vi "pid.vi"(0 "目标":dbl, 1 "当前":dbl, 2 "kp":dbl, 3 "ki":dbl, 4 "kd":dbl, 6 "重置积分":bool) -> (5 "out":dbl)   [LabVIEW 2022 SP3]
panel:
  out "pid微分":dbl
  out "pid积分":dbl
  out "d":dbl
  out "p":dbl
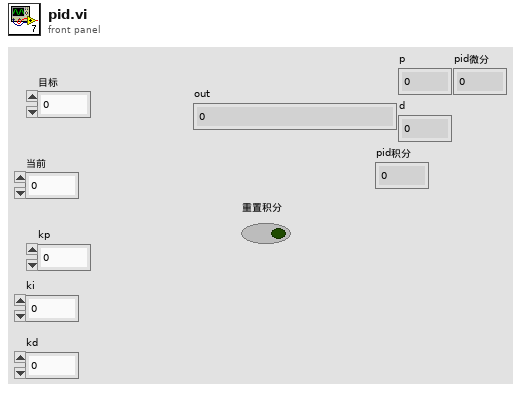
[diagram p1: front panel]
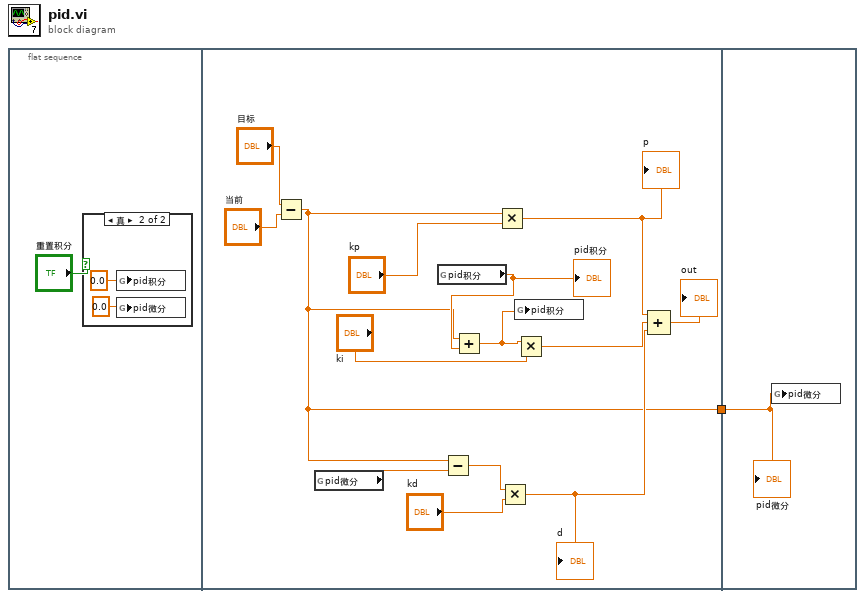
[diagram p0: block diagram]
diagram:
  n1 = flat-sequence {
    tunnel: [w5] -> w1
    tunnel: w1 -> [w19]
    frame #0 {
      n2 = case shown="真" "重置积分" {
        frame False {
        }
        frame True {
          n3 = global write "全局 1.vi" "pid积分"(0.0 ("pid积分")) -> ()
          n4 = global write "全局 1.vi" "pid微分"(0.0 ("pid积分")) -> ()
        }
      }
    }
    frame #1 {
      n5 = Subtract(x="目标", y="当前") -> (x-y=w5:dbl)
      n6 = global read "全局 1.vi" "pid微分"() -> (w6:dbl)
      n7 = global read "全局 1.vi" "pid积分"() -> (w18:dbl)
      "pid积分" <- w18
      n8 = Subtract(x=w5, y=w6) -> (x-y=w11:dbl)
      n9 = Add(x=w5, y=w18) -> (x+y=w17:dbl)
      n10 = Multiply(x=w5, y="kp") -> (x*y=w13:dbl)
      "p" <- w13
      n11 = Multiply(x=w11, y="kd") -> (x*y=w15:dbl)
      "d" <- w15
      n12 = global write "全局 1.vi" "pid积分"(w17) -> ()
      n13 = Multiply(x=w17, y="ki") -> (x*y=w14:dbl)
      n14 = Compound Arithmetic op=ADD(w13, w14, w15) -> (→"out":dbl)
    }
    frame #2 {
      n15 = global write "全局 1.vi" "pid微分"(w19) -> ()
      "pid微分" <- w19
    }
  }
